vi "Build Array Elements.vi"(0 "Elements":u32, 5 "Default Value":dbl, 7 "Units":string, 9 "Name":string, 11 "error in (no error)":errorcluster) -> (4 "Array":T1[](array[typedef]), 15 "error out":errorcluster)   [LabVIEW 2018, in "Instrument Addon System Explorer.lvlib"]
uses:
  Instrument Addon System Explorer.lvlib
  APIs/Scripting API/TypeDefs/Array Element.ctl
  APIs/Scripting API/Instrument Addon Scripting API.lvlib
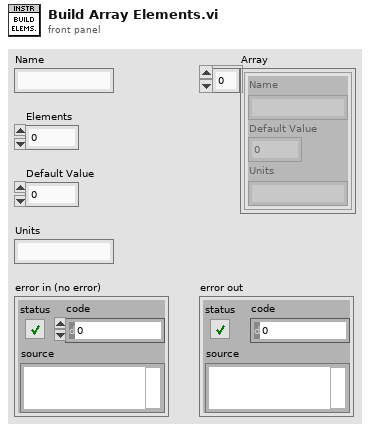
[diagram p1: front panel]
types:
  T1 = typedef "Instrument Addon Scripting API.lvlib/Array Element.ctl" = cluster{"Name":string, "Default Value":dbl, "Units":string}
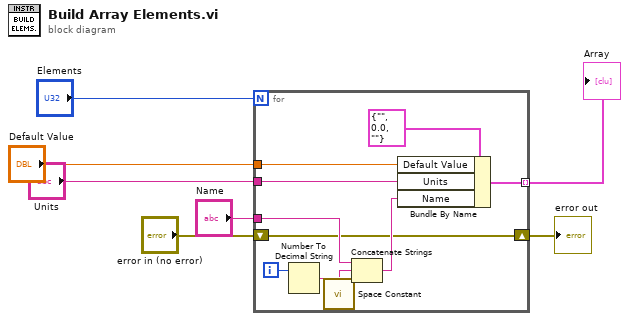
[diagram p0: block diagram]
diagram:
  n1 = for {
    N: "Elements" -> [_]
    shift-right: [w8] -> w6
    shift-left: "error in (no error)" -> [w8]
    tunnel: "Name" -> [w16]
    tunnel: "Units" -> [w13]
    tunnel: "Default Value" -> [w12]
    tunnel: [w9] -> w7 mode=indexing
    i -> [w17]
    n2 = Number To Decimal String(number=w17) -> (decimal integer string=w15:string)  [unwired: 1 in]
    n3 = call <vilib>:"Space Constant.vi"() -> ("String"=w14:string)
    n4 = Concatenate Strings(w16, w14, w15) -> (w10:string)
    n5 = Bundle By Name(cluster=T1 {"Name"="", "Default Value"=0.0, "Units"=""} ("Array Element"), "Default Value"=w12, "Units"=w13, "Name"=w10) -> (w9:T1)
  }
  "Array" <- w7
  "error out" <- w6
